vi "SPC_get_break_time.vi"(8 "Error In":errorcluster, 10 "Module No":i16 min=0 max=7 step=1, 11 "DLL Path":path) -> (0 "Error Out":errorcluster, 2 "Module No":i16 min=0 max=7 step=1, 3 "DLL Path":path, 4 "Time Value":sgl format="%.2f")   [LabVIEW 2017]
doc: "The procedure calculates for the SPC module ‘mod_no’ the time from the start of the measurement to the moment of a measurement interruption by a user break (SPC_stop_measurement or SPC_pause_measurement) or by a stop on overflow.\nThe procedure can be used to find out the moment of measurement interrupt.\n\ninfo@becker-hickl.com"
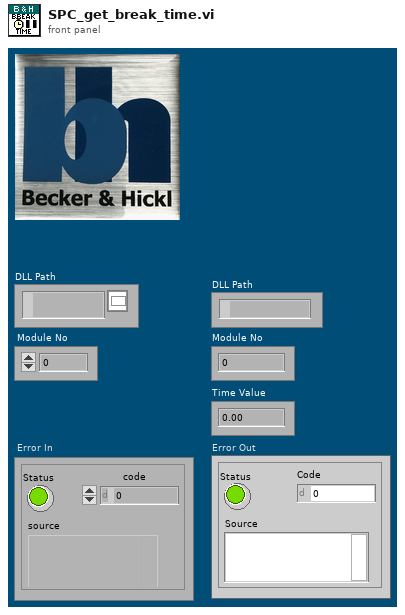
[diagram p1: front panel]
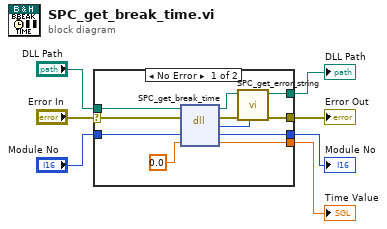
[diagram p0: block diagram]
diagram:
  n1 = case shown="No Error" "Error In" {
    selector: "Error In" -> [w17 w21]
    tunnel: "DLL Path" -> [w18 w20]
    tunnel: [w15 w21] -> w5
    tunnel: [w12 w20] -> w4
    tunnel: [w11 _] -> w3
    tunnel: "Module No" -> [w10 w19]
    tunnel: [w9 w19] -> w1
    frame No Error {
      n2 = dll-call lib="D:/spcm/lib/lab_view/lv10.0/spcm32.dll" fn="SPC_get_break_time"(path in=w18, error in=w17, "mod_no"=w10, "time"=sgl 0.0 ("Last Time Value")) -> (path out=w13:path, error out=w16:errorcluster, "return type"=w14:i16, "mod_no"=w9:i16, "time"=w11:sgl)  [unwired: 1 in]
      n3 = call "SPC_get_error_string.vi"("ErrorID"=w14, "Error In"=w16, "DLL Path"=w13) -> ("Error Out"=w15:errorcluster, "DLL Path"=w12:path)  [unwired: 6 in, 1 out]
    }
    frame Error {
    }
  }
  "DLL Path" <- w4
  "Error Out" <- w5
  "Time Value" <- w3
  "Module No" <- w1
